vi "CIF Waveform to DVR.vi"(7 "gRPC Waveform Enabled":bool, 8 "error in (no error)":errorcluster, 10 "CIF Waveforms in":T1[](array[typedef]), 11 "gRPC Waveform Monitor in":T2) -> (0 "error out":errorcluster, 2 "CIF Waveforms out":T1[](array[typedef]), 3 "gRPC Waveform Monitor out":T2)   [LabVIEW 2021, in "CIFWaveformMonitorWrapper.lvlib"]
uses:
  CIFWaveformMonitorWrapper.lvlib
  Typedef/CIF Wave Array DVR.ctl
  <vilib>/CIF Foundation/CIF Channels Core/ChannelCommon/typedef/Datatype Waveform.ctl
  <vilib>/CIF Foundation/CIF Channels Core/ChannelCommon/ChannelCommon.lvlib
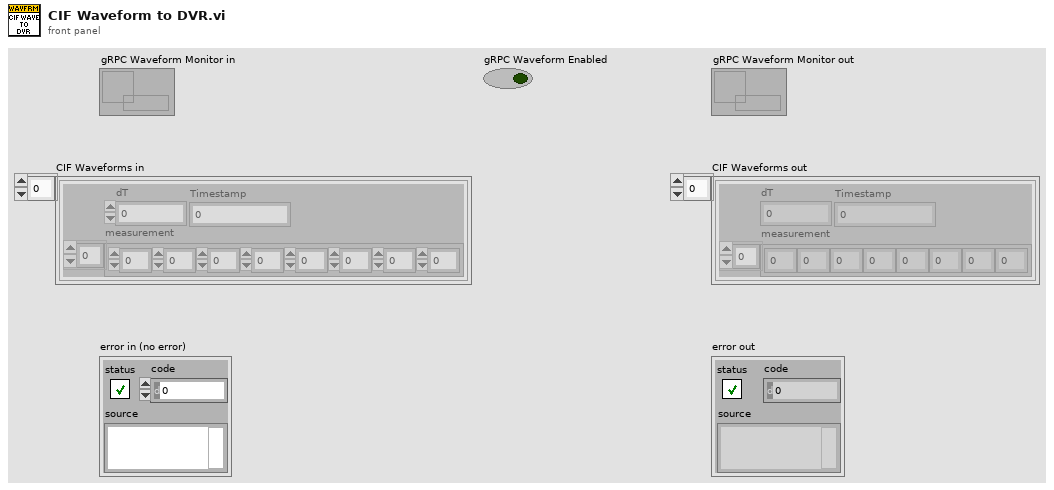
[diagram p1: front panel]
types:
  T1 = typedef "ChannelCommon.lvlib/Datatype Waveform.ctl" = cluster{"measurement":dbl[], "dT":dbl, "Timestamp":i64}
  T2 = typedef "CIFWaveformMonitorWrapper.lvlib/CIF Wave Array DVR.ctl" = refnum<data-value>
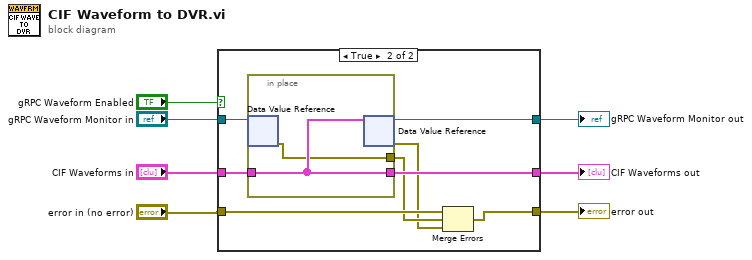
[diagram p0: block diagram]
diagram:
  n1 = case shown="True" "gRPC Waveform Enabled" {
    tunnel: "gRPC Waveform Monitor in" -> [w8 w18]
    tunnel: "CIF Waveforms in" -> [w10 w17]
    tunnel: [w10 w16] -> w1
    tunnel: "error in (no error)" -> [w9 w15]
    tunnel: [w9 w12] -> w6
    tunnel: [w8 w11] -> w4
    frame False {
    }
    frame True {
      n2 = in-place {
        in-place-border: w17 -> [w20]
        in-place-border: [w20] -> w16
        in-place-border: [w19] -> w14
        n3 = in-place-dvr #1(w18) -> (w19:errorcluster)  [unwired: 1 out]
        n4 = in-place-dvr #1(w20) -> (w11:T2, w13:errorcluster)
      }
      n5 = Merge Errors(w15, w14, w13) -> (w12:errorcluster)
    }
  }
  "error out" <- w6
  "gRPC Waveform Monitor out" <- w4
  "CIF Waveforms out" <- w1
